vi "Test Check Keys.vi"() -> ()   [LabVIEW 2012]
panel:
  in  "Time Stamp 3":timestamp
  in  "Time Stamp 2":timestamp
  in  "Time Stamp":timestamp
  in  "Time":timestamp
  out "Sorted Data Out":T1
  out "codelapse":bool
  in  "Sorted Data in":T1
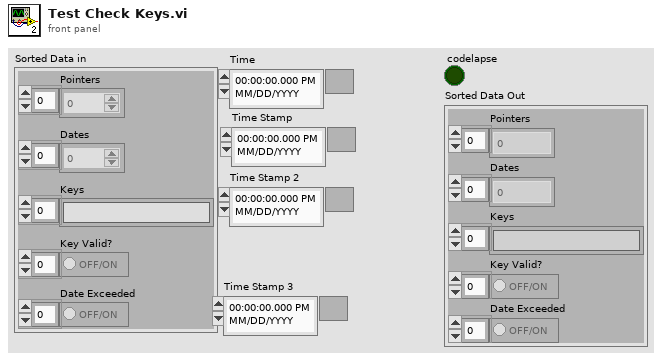
[diagram p1: front panel]
types:
  T1 = cluster{"Pointers":i32[], "Dates":dbl[], "Keys":string[], "Key Valid?":bool[], "Date Exceeded":bool[]}
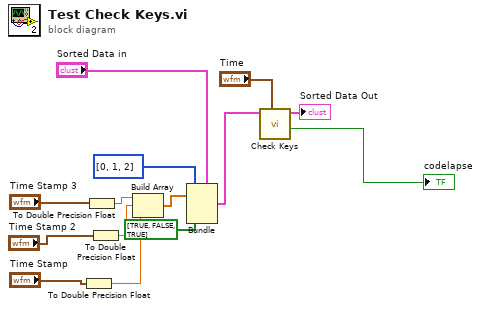
[diagram p0: block diagram]
diagram:
  n1 = To Double Precision Float(number="Time Stamp") -> (double precision float=w6:dbl)
  n2 = To Double Precision Float(number="Time Stamp 3") -> (double precision float=w8:dbl)
  n3 = To Double Precision Float(number="Time Stamp 2") -> (double precision float=w7:dbl)
  n4 = Build Array(w8, w7, w6) -> (w3:dbl[])
  n5 = Bundle(cluster="Sorted Data in", "Pointers"=i32[] [0, 1, 2], "Dates"=w3, "Key Valid?"=bool[] [TRUE, FALSE, TRUE]) -> (w1:T1)  [unwired: 2 in]
  n6 = call "Check Keys.vi"("Time"="Time", "Sorted Data in"=w1) -> ("codelapse"=→"codelapse":bool, "Sorted Data Out"=→"Sorted Data Out":T1)  [unwired: 8 in]
